vi "Handle Parameter 3 Control.vi"(0 "Reference In":refnum<vi>, 2 "Mode":enum16{"Init", "Set"}(ring)=enum."Set", 5 "Parameter 1":i32, 7 "Parameter 2":i32, 9 "Stop Command":dbl format="%#_13g", 11 "Last Command":dbl format="%#_13g", 12 "Error In":errorcluster) -> (6 "Parameter 3":i32, 10 "Command  Out":dbl format="%#_13g", 15 "Error Out":errorcluster)   [LabVIEW 2013]
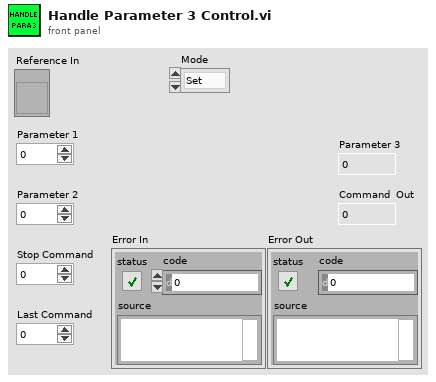
[diagram p1: front panel]
types:
  T1 = enum16{"Voltage", "Pressure", "Flow", "Speed", "Duty Cycle"}
  T2 = enum16{"Voltage", "Pressure", "Flow", "Speed", "Command"}
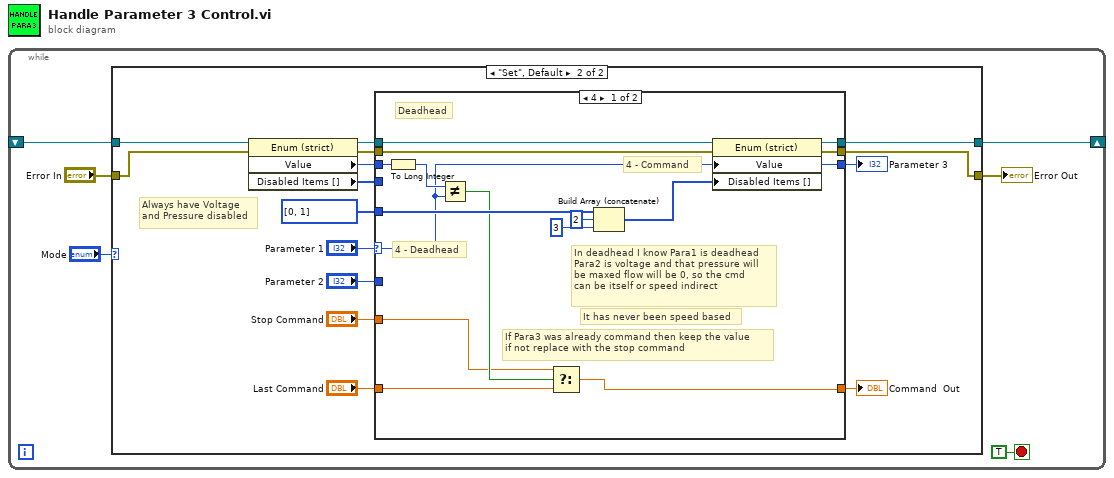
[diagram p0: block diagram]
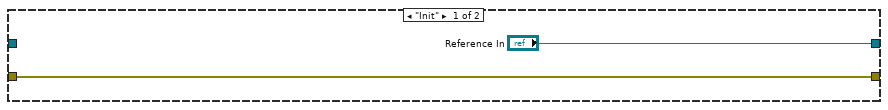
[diagram p2: hidden frame]
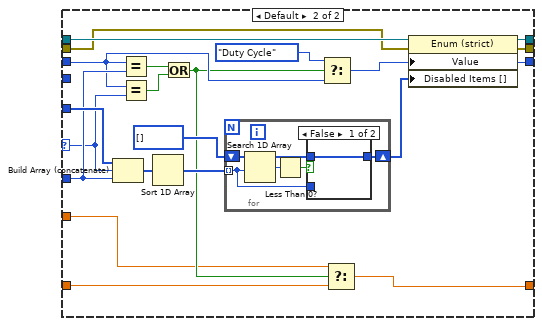
[diagram p3: hidden frame]
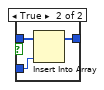
[diagram p4: hidden frame]
diagram:
  n1 = while {
    shift-right: [w4] -> _
    shift-left: _ -> [w3]
    stop <- TRUE stop-if-true
    n2 = case shown="\"Set\", Default" "Mode" {
      tunnel: w3 -> [_ w12]
      tunnel: ["Reference In" w13] -> w4
      tunnel: "Error In" -> [w7 w11]
      tunnel: [w7 w9] -> w1
      frame "Init" {
      }
      frame "Set", Default {
        # "Always have Voltage\nand Pressure disabled"
        n3 = property class="Enum (strict)"(reference=w12, error in=w11) -> (reference out=w16:refnum<vi>, error out=w10:errorcluster, "Value"=w15:T2, "Disabled Items []"=w14:i32[])
        n4 = case shown="4" "Parameter 1" {
          selector: "Parameter 1" -> [w29 w53]
          tunnel: w15 -> [w31 w50]
          tunnel: w14 -> [_ _]
          tunnel: "Parameter 2" -> [_ w54]
          tunnel: "Stop Command" -> [w26 w47]
          tunnel: w16 -> [w37 w44]
          tunnel: i32[] [0, 1] -> [w38 w58]
          tunnel: "Last Command" -> [w25 w46]
          tunnel: [w27 w45] -> w18
          tunnel: [w29 w43] -> w17
          tunnel: [w36 w41] -> w13
          tunnel: w10 -> [w35 w40]
          tunnel: [w34 w39] -> w9
          frame 4 {
            # "It has never been speed based"
            # "If Para3 was already command then keep the value\nif not replace with the stop command"
            # "4 - Command"
            # "4 - Deadhead"
            # "In deadhead I know Para1 is deadhead\nPara2 is voltage and that pressure will\nbe maxed flow will be 0, so the cmd\ncan be itself or speed indirect"
            # "Deadhead"
            n5 = To Long Integer(number=w31) -> (32bit integer=w30:i32)
            n6 = Not Equal?(x=w30, y=w29) -> (x != y?=w28:bool)
            n7 = Select(t=w26, s=w28, f=w25) -> (s? t:f=w27:dbl)
            n8 = Build Array (concatenate)(w38, 2, 3) -> (w32:i32[])
            n9 = property class="Enum (strict)"(reference=w37, error in=w35, "Value"=w29, "Disabled Items []"=w32) -> (reference out=w36:refnum<vi>, error out=w34:errorcluster)
          }
          frame Default {
            n10 = Build Array (concatenate)(w58, w53, w54) -> (w57:i32[])
            n11 = Equal?(x=w50, y=w54) -> (x = y?=w52:bool)
            n12 = Equal?(x=w50, y=w53) -> (x = y?=w51:bool)
            n13 = Sort 1D Array(array=w57) -> (sorted array=w56:i32[])
            n14 = Or(x=w52, y=w51) -> (x .or. y?=w48:bool)
            n15 = for {
              tunnel: w56 -> [w59] mode=indexing
              shift-right: [w60] -> w42
              shift-left: i32[] [] -> [w61]
              n16 = Search 1D Array(1D array=w61, element=w59) -> (index of element=w63:i32)  [unwired: 1 in]
              n17 = Less Than 0?(x=w63) -> (x < 0?=w62:bool)
              n18 = case shown="False" w62 {
                tunnel: w61 -> [w64 w67]
                tunnel: [w64 w66] -> w60
                tunnel: w59 -> [_ w65]
                frame False {
                }
                frame True {
                  n19 = Insert Into Array(array=w67, new element=w65) -> (w66:i32[])  [unwired: 1 in]
                }
              }
            }
            n20 = Select(t=T1."Duty Cycle", s=w48, f=w50) -> (s? t:f=w43:u16)
            n21 = Select(t=w47, s=w48, f=w46) -> (s? t:f=w45:dbl)
            n22 = property class="Enum (strict)"(reference=w44, error in=w40, "Value"=w43, "Disabled Items []"=w42) -> (reference out=w41:refnum<vi>, error out=w39:errorcluster)
          }
        }
        "Command  Out" <- w18
        "Parameter 3" <- w17
      }
    }
    "Error Out" <- w1
  }
